vi "Reset.vi"(11 "Hash Function in":refnum<class "NI_SHA-3.lvclass">) -> (3 "Hash Function out":refnum<class "NI_SHA-3.lvclass">)   [LabVIEW 2020, in "NI_SHA-3.lvclass"]
uses:
  <vilib>/security/Message Digest/SHA-3/NI_SHA-3.lvclass
  <vilib>/security/Message Digest/SHA-3/subVIs/state.ctl
  <vilib>/security/Message Digest/SHA-3/subVIs/state word.ctl
  <vilib>/security/Message Digest/SHA-3/NI_SHA-3.lvclass/NI_SHA-3.ctl
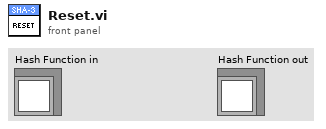
[diagram p1: front panel]
types:
  T1 = typedef "NI_SHA-3.lvclass/state.ctl" = cluster{"A00":T2, "A01":T2, "A02":T2, "A03":T2, "A04":T2, "A05":T2, "A06":T2, "A07":T2, "A08":T2, "A09":T2, "A10":T2, "A11":T2, "A12":T2, "A13":T2, "A14":T2, "A15":T2, "A16":T2, "A17":T2, "A18":T2, "A19":T2, "A20":T2, "A21":T2, "A22":T2, "A23":T2, "A24":T2}
  T2 = typedef "NI_SHA-3.lvclass/state word.ctl" = u64
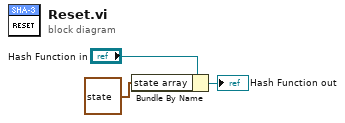
[diagram p0: block diagram]
diagram:
  n1 = Bundle By Name(cluster="Hash Function in", "state array"=T1 {"A00"=0, "A01"=0, "A02"=0, "A03"=0, "A04"=0, "A05"=0, "A06"=0, "A07"=0, "A08"=0, "A09"=0, "A10"=0, "A11"=0, "A12"=0, "A13"=0, "A14"=0, "A15"=0, "A16"=0, "A17"=0, "A18"=0, "A19"=0, "A20"=0, "A21"=0, "A22"=0, "A23"=0, "A24"=0}) -> (→"Hash Function out":refnum<class "NI_SHA-3.lvclass">)
